vi "TimingTest.vi"() -> ()   [LabVIEW 2016]
uses:
  <vilib>/FPGAPlugInAG/cRIO-9038/niLvFpga_Open_cRIO-9038.vi
  <vilib>/rvi/interface/common/dynamic/niFpgaDynamicAddResources.vi
  <vilib>/FPGAPlugInAG/Dynamic/niLvFpga_Abort_Dynamic.vi
  <vilib>/FPGAPlugInAG/Dynamic/niLvFpga_Reset_Dynamic.vi
  <vilib>/FPGAPlugInAG/Dynamic/niLvFpga_Run_Dynamic.vi
  <vilib>/Utility/error.llb/Error Cluster From Error Code.vi
  <vilib>/rvi/errors/niLvFpgaAdjustHostInterfaceError.vi
  <vilib>/FPGAPlugInAG/Dynamic/niLvFpga_Close_Dynamic.vi
  <vilib>/rvi/interface/nirviOpenFPGA/nirviOpenFPGA.xnode
  FPGA Bitfiles/modbus1Port.lvbitx
  FPGA/main.vi
  <vilib>/rvi/interface/nirviMethod/nirviMethod.xnode
  <vilib>/rvi/interface/nirviCloseFPGA/nirviCloseFPGA.xnode
  <vilib>/rvi/errors/niLvFpgaMergeErrorWithErrorCode.vi
  <vilib>/FPGAPlugInAG/Dynamic/niLvFpga_ReadFifo_Dynamic.vi
  <vilib>/FPGAPlugInAG/Dynamic/niLvFpga_WriteFifo_Dynamic.vi
panel:
  in  "Boolean":bool
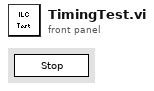
[diagram p1: front panel]
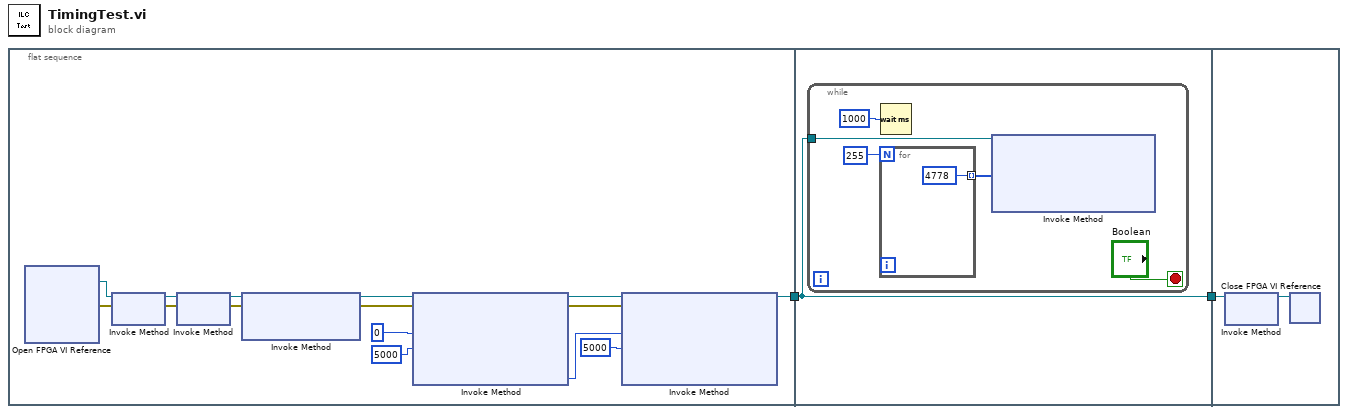
[diagram p0: block diagram]
diagram:
  n1 = flat-sequence {
    tunnel: [w6] -> w2
    tunnel: w2 -> [w18]
    tunnel: [w18] -> w1
    tunnel: w1 -> [w25]
    frame #0 {
      n2 = xnode "Open FPGA VI Reference"() -> ("FPGA VI Reference Out"=w15:refnum<k20>, "error out"=w3:errorcluster)  [unwired: 2 in]
      n3 = xnode "Invoke Method"("FPGA VI Reference In"=w15, "error in"=w3) -> ("FPGA VI Reference Out"=w17:refnum<k20>, "error out"=w16:errorcluster)
      n4 = xnode "Invoke Method"("FPGA VI Reference In"=w17, "error in"=w16) -> ("FPGA VI Reference Out"=w8:refnum<k20>, "error out"=w5:errorcluster)
      n5 = xnode "Invoke Method"("FPGA VI Reference In"=w8, "error in"=w5) -> ("FPGA VI Reference Out"=w7:refnum<k20>, "error out"=w4:errorcluster)  [unwired: 1 in]
      n6 = xnode "Invoke Method"("FPGA VI Reference In"=w7, "error in"=w4, "Number of Elements"=u32 0, "Timeout (ms)"=5000) -> ("FPGA VI Reference Out"=w11:refnum<k20>, "error out"=w9:errorcluster, "Elements Remaining"=w12:u32)  [unwired: 1 out]
      n7 = xnode "Invoke Method"("FPGA VI Reference In"=w11, "error in"=w9, "Number of Elements"=w12, "Timeout (ms)"=5000) -> ("FPGA VI Reference Out"=w6:refnum<k20>)  [unwired: 3 out]
    }
    frame #1 {
      n8 = while {
        tunnel: w18 -> [w22]
        stop <- "Boolean" stop-if-true
        n9 = for {
          N: 255 -> [_]
          tunnel: [u16 4778 ("x")] -> w20 mode=indexing
        }
        n10 = Wait (ms)(milliseconds to wait=u32 1000) -> ()  [unwired: 1 out]
        n11 = xnode "Invoke Method"("FPGA VI Reference In"=w22, "Data"=w20) -> ()  [unwired: 2 in, 3 out]
      }
    }
    frame #2 {
      n12 = xnode "Invoke Method"("FPGA VI Reference In"=w25) -> ("FPGA VI Reference Out"=w26:refnum<k20>)  [unwired: 1 in, 1 out]
      n13 = xnode "Close FPGA VI Reference"("FPGA VI Reference In"=w26) -> ()  [unwired: 1 in, 1 out]
    }
  }
